vi "test refnum.vi"(11 "LTS Reference":refnum<k24>(container)) -> (3 "LTS Reference 2":refnum<k24>(container))   [LabVIEW 2018]
uses:
  C:/Project/SerialSectionOCT/SerialSectOCT/Labview Software/Thorlabs.MotionControl.Controls.dll
  Thorlabs.MotionControl.Controls.dll
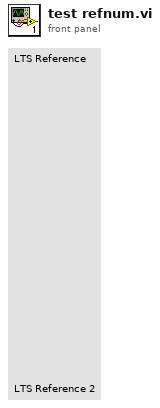
[diagram p1: front panel]
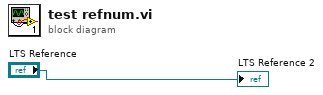
[diagram p0: block diagram]
diagram:
  "LTS Reference 2" <- "LTS Reference"
